vi "CheckUnload.vi"(8 "error in (no error)":errorcluster, 11 "EpiWrapper in":refnum<class "EpiWrapper.lvclass">) -> (0 "error out":errorcluster, 2 "Continue":bool, 3 "EpiWrapper out":refnum<class "EpiWrapper.lvclass">)   [LabVIEW 2012, in "EpiWrapper.lvclass"]
uses:
  EpiWrapper.lvclass
  EpiWrapper.lvclass/EpiWrapper.ctl
  LotData.lvclass
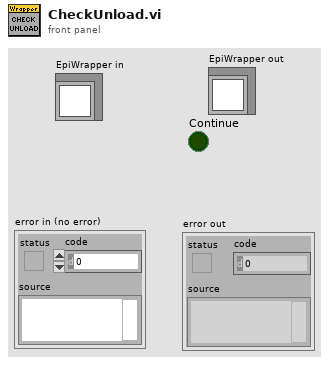
[diagram p1: front panel]
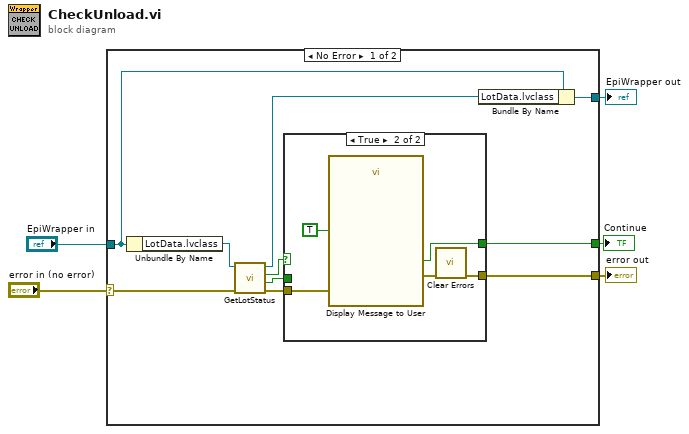
[diagram p0: block diagram]
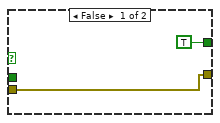
[diagram p2: hidden frame]
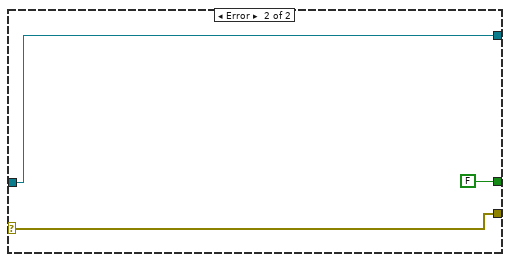
[diagram p3: hidden frame]
diagram:
  n1 = case shown="No Error" "error in (no error)" {
    selector: "error in (no error)" -> [w14 w25]
    tunnel: [w11 w25] -> w4
    tunnel: [w6 w24] -> w2
    tunnel: "EpiWrapper in" -> [w8 w24]
    tunnel: [w9 FALSE ("Continue")] -> w1
    frame No Error {
      n2 = Unbundle By Name(w8) -> ("LotData.lvclass"=w15:refnum<class "LotData.lvclass">)
      n3 = call-dynamic "GetLotStatus.vi"("error in (no error)"=w14, "LotData in"=w15) -> ("error out"=w10:errorcluster, "Saved"=w12:bool, "Loaded"=w13:bool, "LotData out"=w7:refnum<class "LotData.lvclass">)  [unwired: 6 in]
      n4 = case shown="True" w13 {
        tunnel: w12 -> [_ _]
        tunnel: [w16 w20] -> w11
        tunnel: w10 -> [w16 w19]
        tunnel: [TRUE ("Continue") w18] -> w9
        frame False {
        }
        frame True {
          n5 = call "Display Message to User"("error in (no error)"=w19, "Enable"=TRUE) -> ("error out"=w22:errorcluster, "Continue"=w18:bool)  [unwired: 8 in]
          n6 = call <vilib>:"Clear Errors.vi"("error in (no error)"=w22) -> ("error out"=w20:errorcluster)  [unwired: 6 in]
        }
      }
      n7 = Bundle By Name(cluster=w8, "LotData.lvclass"=w7) -> (w6:refnum<class "EpiWrapper.lvclass">)
    }
    frame Error {
    }
  }
  "error out" <- w4
  "EpiWrapper out" <- w2
  "Continue" <- w1
